vi "PH_SHS_Analysis_Statistician.export Data.vi"(0 "i ref in":refnum<vi>, 5 "error in (no error)":errorcluster) -> (14 "i ref out":refnum<vi>, 19 "error out":errorcluster)   [LabVIEW 2014, in "PH_SHS_Analysis_Statistician.lvlib"]
doc: "This VI exports data to a file"
uses:
  PH_SHS_Analysis_Statistician.lvlib
  PH_Common/PH_Common.lvlib
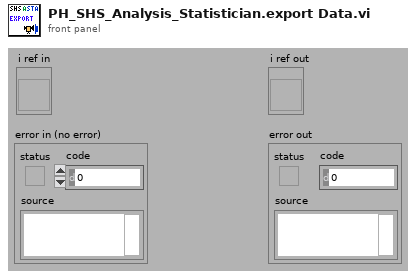
[diagram p1: front panel]
types:
  T1 = typedef "PH_SHS_Analysis_Statistician.lvlib/PH_SHS_Analysis_Statistician.i attribute.ctl" = cluster{"GUI Refs ":cluster{"Status":refnum<vi>, "Result Graph":refnum<vi>, "Mean Data 1":refnum<vi>, "Std Dev Data 1":refnum<vi>, "Mean Data 2":refnum<vi>, "Std Dev Data 2":refnum<vi>, "Mean Data 3":refnum<vi>, "Std Dev Data 3":refnum<vi>, "Dummy Mean":refnum<vi>, "Dummy Std Dev":refnum<vi>, "Export Data":refnum<vi>, "Data 1":refnum<vi>, "Data 2":refnum<vi>, "Data 3":refnum<vi>, "Stat or Trend":refnum<vi>, "Delete":refnum<vi>, "Analyzer":refnum<vi>, "Current Zernike Coefficients":refnum<vi>, "PtV [Lambda]":refnum<vi>, "sample length":refnum<vi>}, "Analyzer":string, "Stat or Trend":bool, "Data 1":i16, "Data 2":i16, "Data 3":i16, "Data":T2[], "sample length":i32, "Datasets strored":i32, "Dataarray Size":i32}
  T2 = typedef "PH_SHS_Analysis.lvlib/PH_SHS_Analysis.Zernike Dataset.ctl" = cluster{"State":T3, "Time Stamp":timestamp, "PtV [lambda]":dbl, "Zernicke Coefficients":T4}
  T3 = typedef "PH_StatusHandler.lvlib/PH_StatusHandler.Status.ctl" = i16
  T4 = typedef "PH_SHS_Analysis.lvlib/PH_SHS_Analysis.Zernike Coefficients.ctl" = cluster{"Tilt x":dbl, "Tilt y":dbl, "Defocus":dbl, "Astig 0°":dbl, "Astig 45°":dbl, "Coma x":dbl, "Coma y":dbl, "Spherical":dbl, "Trefoil 0°":dbl, "Trefoil 30°":dbl, "2nd Astig 0°":dbl, "2nd Astig 45°":dbl, "2nd Coma x":dbl, "2nd Coma y":dbl, "2nd Spherical":dbl}
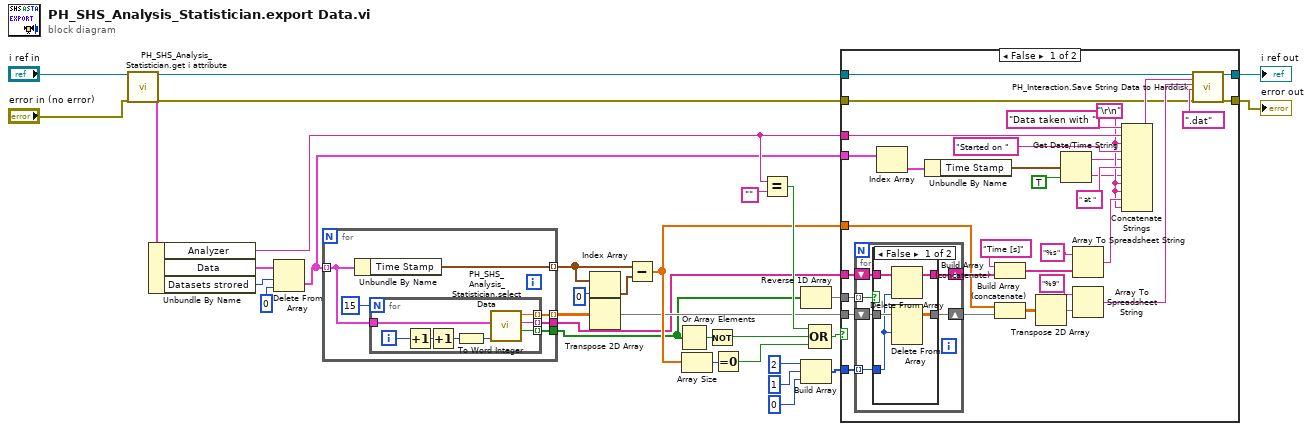
[diagram p0: block diagram]
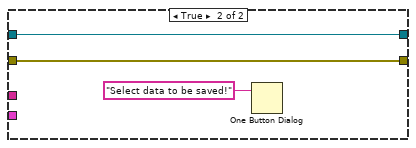
[diagram p3: hidden frame]
diagram:
  n1 = call "PH_SHS_Analysis_Statistician.get i attribute.vi"("i ref in"="i ref in", "error in (no error)"="error in (no error)") -> ("i ref out"=w5:refnum<vi>, "i attribute"=w18:T1, "error out"=w6:errorcluster)  [unwired: 15 in]
  n2 = Unbundle By Name(w18) -> ("Analyzer"=w7:string, "Data"=w4:T2[], "Datasets strored"=w2:i32)
  n3 = Delete From Array(array=w4, length=w2, index=0) -> (deleted portion=w3:T2[])  [unwired: 1 out]
  n4 = for {
    tunnel: w3 -> [w38] mode=indexing
    tunnel: [w34] -> w16 mode=indexing
    tunnel: [w37] -> w11
    tunnel: [w36] -> w10
    tunnel: [w35] -> w17 mode=indexing
    n5 = Unbundle By Name(w38) -> ("Time Stamp"=w34:timestamp)
    n6 = for {
      N: 15 -> [_]
      tunnel: w38 -> [w43]
      tunnel: [w46] -> w37 mode=indexing
      tunnel: [w45] -> w36 mode=indexing
      tunnel: [w44] -> w35 mode=indexing
      i -> [w42]
      n7 = Increment(x=w42) -> (x+1=w39:i32)
      n8 = Increment(x=w39) -> (x+1=w41:i32)
      n9 = To Word Integer(number=w41) -> (16bit integer=w40:i16)
      n10 = call "PH_SHS_Analysis_Statistician.select Data.vi"("Data Selector"=w40, "SHS Analyzer Dataset"=w43) -> ("Data chosen?"=w45:bool, "Data Legend"=w46:string, "Data"=w44:dbl)  [unwired: 5 in]
    }
  }
  n11 = Index Array(array=w16, index=0) -> (element=w14:timestamp)
  n12 = Transpose 2D Array(2D array=w17) -> (transposed array=w12:dbl[][])
  n13 = Subtract(x=w16, y=w14) -> (x-y=w13:dbl[])
  n14 = Or Array Elements(Boolean array=w10) -> (logical OR=w29:bool)
  n15 = Array Size(array=w13) -> (size(s)=w25:i32)
  n16 = Not(x=w29) -> (.not. x?=w28:bool)
  n17 = Equal To 0?(x=w25) -> (x = 0?=w24:bool)
  n18 = Equal?(x=w7, y="") -> (x = y?=w27:bool)
  n19 = Reverse 1D Array(array=w10) -> (reversed array=w19:bool[])
  n20 = Build Array(2, 1, 0) -> (w20:i32[])
  n21 = Compound Arithmetic op=OR(w27, w28, w24) -> (w26:bool)
  n22 = case shown="False" w26 {
    tunnel: w7 -> [w74 _]
    tunnel: w11 -> [w70 _]
    tunnel: w12 -> [w68 _]
    tunnel: w19 -> [w69 _]
    tunnel: w6 -> [w56 w93]
    tunnel: [w55 w93] -> w32
    tunnel: w13 -> [w64 _]
    tunnel: w20 -> [w61 _]
    tunnel: w5 -> [w54 w92]
    tunnel: [w53 w92] -> w31
    tunnel: w3 -> [w48 _]
    frame False {
      w71 = "\r\n"
      n23 = for {
        tunnel: w69 -> [w80] mode=indexing
        shift-right: [w83] -> w66
        shift-left: w70 -> [w84]
        shift-right: [w81] -> w63
        shift-left: w68 -> [w82]
        tunnel: w61 -> [w79] mode=indexing
        n24 = case shown="False" w80 {
          tunnel: w84 -> [w89 w91]
          tunnel: [w88 w91] -> w83
          tunnel: w82 -> [w87 w90]
          tunnel: [w86 w90] -> w81
          tunnel: w79 -> [w85 _]
          frame False {
            n25 = Delete From Array(array=w89, index=w85) -> (array with subset deleted=w88:string[])  [unwired: 1 in, 1 out]
            n26 = Delete From Array(array=w87, index (row)=w85) -> (array with subset deleted=w86:dbl[][])  [unwired: 2 in, 1 out]
          }
          frame True {
          }
        }
      }
      n27 = Index Array(array=w48) -> (element=w49:T2)  [unwired: 1 in]
      n28 = Unbundle By Name(w49) -> ("Time Stamp"=w47:timestamp)
      n29 = Build Array (concatenate)("Time [s]" ("element"), w66) -> (w65:string[])
      n30 = Build Array (concatenate)(w64, w63) -> (w62:dbl[][])
      n31 = Transpose 2D Array(2D array=w62) -> (transposed array=w67:dbl[][])
      n32 = Get Date/Time String(seconds (now)=w47, want seconds? (F)=TRUE) -> (date string=w51:string, time string=w50:string)  [unwired: 1 in]
      n33 = Array To Spreadsheet String(array=w65, 3:"%s" ("format string")) -> (spreadsheet string=w72:string)  [unwired: 1 in]
      n34 = Array To Spreadsheet String(array=w67, 3:"%9" ("format string")) -> (spreadsheet string=w59:string)  [unwired: 1 in]
      n35 = Concatenate Strings("Data taken with " ("string"), w74, w71, "Started on ", w51, " at " ("string"), w50, w71, w71, w72, w71) -> (w57:string)
      n36 = call "PH_Interaction.Save String Data to Harddisk.vi"("i ref in"=w54, "Explanation (for Example: Column 1: xxx, ...)"=w57, "Data (for example: Columns)"=w59, "file name extension"=".dat" ("file name extinction"), "error in (no error)"=w56) -> ("i ref out"=w53:refnum<vi>, "error out"=w55:errorcluster)  [unwired: 12 in, 1 out]
    }
    frame True {
      n37 = One Button Dialog(message="Select data to be saved!") -> ()  [unwired: 1 in, 1 out]
    }
  }
  "error out" <- w32
  "i ref out" <- w31
